vi "Read states.vi"(8 "error in (no error)":errorcluster, 11 "SupportAttackerRole in":refnum<class "SupportAttackerRole.lvclass">) -> (0 "error out":errorcluster, 2 "States":T1, 3 "SupportAttackerRole out":refnum<class "SupportAttackerRole.lvclass">)   [LabVIEW 2023, in "SupportAttackerRole.lvclass"]
uses:
  SupportAttackerRole.lvclass
  SupportAttackerRole_states.ctl
  SupportAttackerRole.lvclass/SupportAttackerRole.ctl
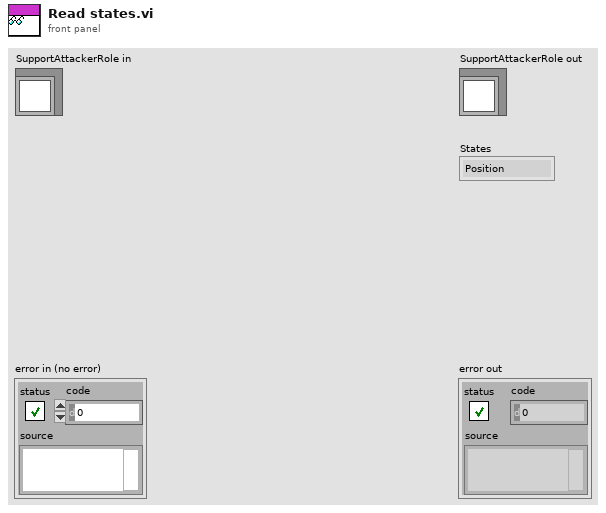
[diagram p1: front panel]
types:
  T1 = typedef "SupportAttackerRole.lvclass/SupportAttackerRole_states.ctl" = enum16{"Position", "WaitPass", "Exit"}
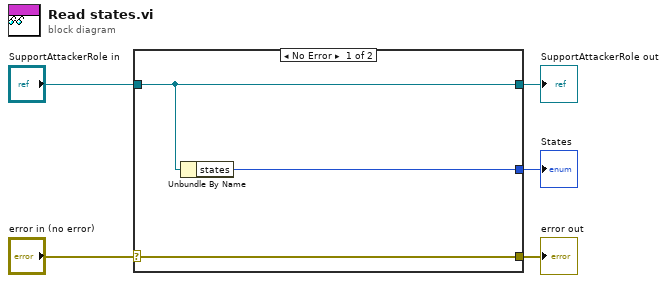
[diagram p0: block diagram]
diagram:
  n1 = case shown="No Error" "error in (no error)" {
    selector: "error in (no error)" -> [w8 w9]
    tunnel: [w8 w9] -> w4
    tunnel: [w7 w10] -> w2
    tunnel: "SupportAttackerRole in" -> [w7 w10]
    tunnel: [w6 _] -> w1
    frame No Error {
      n2 = Unbundle By Name(w7) -> ("states"=w6:T1)
    }
    frame Error {
    }
  }
  "error out" <- w4
  "SupportAttackerRole out" <- w2
  "States" <- w1
